vi "stop while loop_demoinfocom.vi"() -> (3 "Boolean":bool)   [LabVIEW 2021]
uses:
  system stop.vi
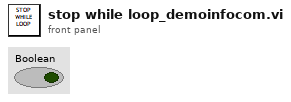
[diagram p1: front panel]
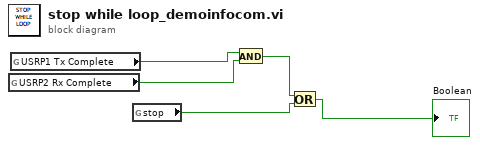
[diagram p0: block diagram]
diagram:
  n1 = global read "system stop.vi" "USRP2 Rx Complete"() -> (w3:bool)
  n2 = global read "system stop.vi" "USRP1 Tx Complete"() -> (w5:bool)
  n3 = global read "system stop.vi" "stop"() -> (w1:bool)
  n4 = And(x=w5, y=w3) -> (x .and. y?=w4:bool)
  n5 = Or(x=w4, y=w1) -> (x .or. y?=→"Boolean":bool)
